vi "tc_array.vi"(0 "String":string, 1 "Numeric":dbl format="%#_13g", 2 "Color Box":u32(colorbox)=4250624, 3 "index (row)":i32, 4 "output array 2":T1(array[cluster]), 5 "PlotColor":u32(colorbox)=16860) -> (6 "output array":T1(array[cluster]) {"Numeric" format="%#.2g"})   [LabVIEW 2016]
panel:
  in  "index (col)":i32
  out "Cluster":T2
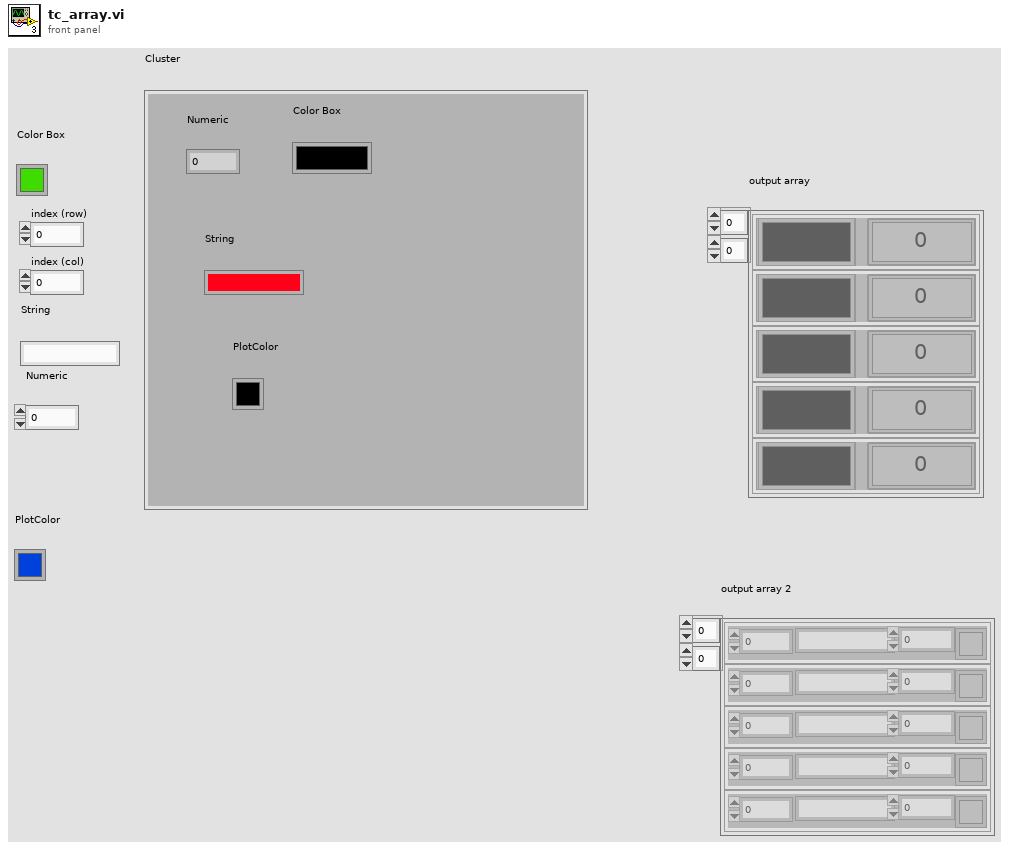
[diagram p1: front panel]
types:
  T1 = cluster{"Numeric":dbl, "Color Box":u32, "String":string, "PlotColor":u32}[][]
  T2 = cluster{"Numeric":dbl, "Color Box":u32, "String":string, "PlotColor":u32}
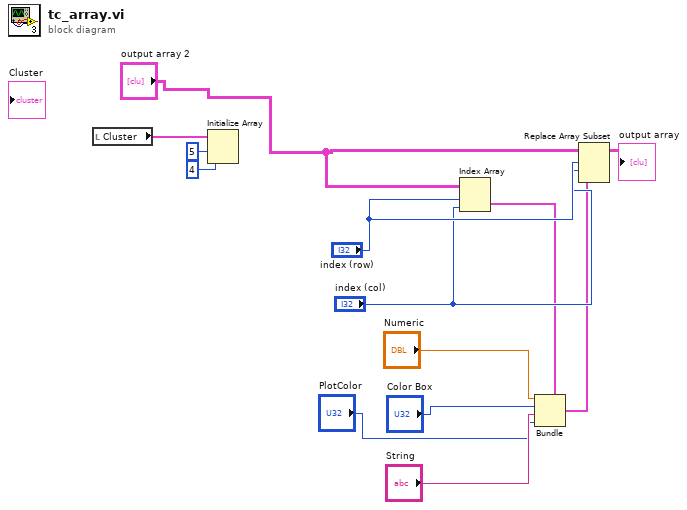
[diagram p0: block diagram]
diagram:
  n1 = local read "Cluster"() -> (w11:T2)
  n2 = Initialize Array(w11, 5 ("dimension size"), 4 ("dimension size")) -> ()  [unwired: 1 out]
  n3 = Index Array(array="output array 2", index (row)="index (row)", index (col)="index (col)") -> (element=w5:T2)
  n4 = Bundle(cluster=w5, "Numeric"="Numeric", "Color Box"="Color Box", "String"="String", "PlotColor"="PlotColor") -> (w6:T2)
  n5 = Replace Array Subset(array="output array 2", new element=w6, index (row)="index (row)", index (col)="index (col)") -> (→"output array":T1)
